vi "RT Loop - Acquire camera_data.vi"(11 "Message Queue":refnum<queue>) -> (3 "Refnum out":T1(plugin-control))   [LabVIEW 2017]
uses:
  UI Error Handlers/support/Message Queue/Message Cluster.ctl
  <vilib>/userdefined/High Color/IMAQdx.ctl
  <vilib>/vision/Avi.llb/IMAQ AVI2 Codec Path.ctl
  <vilib>/vision/Avi.llb/IMAQ AVI2 Refnum.ctl
  Globals/Global - All RT Loop Stop.vi
  Globals/Global - Configuration Options.vi
  <vilib>/vision/driver/NI_Vision_Acquisition_Software.lvlib
  UI Error Handlers/support/Message Queue/Message Queue.lvlib
panel:
  out "Acceleration Log Folder":path=path "/home/lvuser/Log/logfiles_deploy"
  out "Codec Names":string[](array[string])
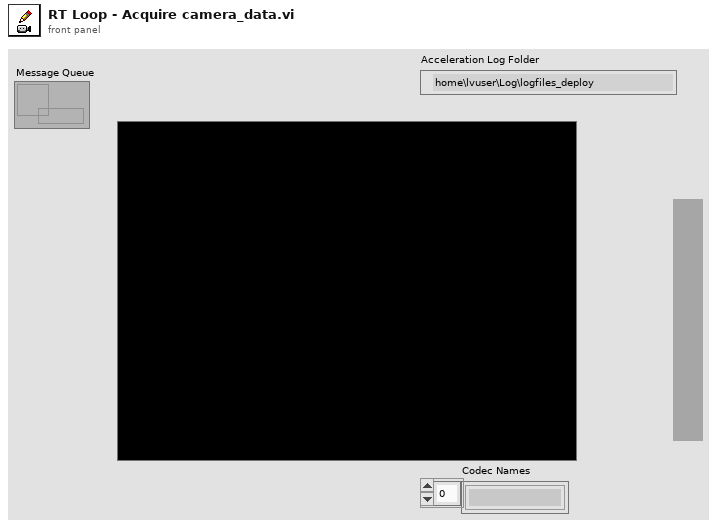
[diagram p1: front panel]
types:
  T1 = typedef "IMAQ Image.ctl" = refnum<image>
  T2 = typedef "IMAQdx.ctl" = refnum<k21>
  T3 = typedef "Image Type" = u32
  T4 = typedef "IMAQ AVI2 Refnum.ctl" = refnum<k20>
  T5 = typedef "IMAQ AVI2 Codec Path.ctl" = u32
  T6 = cluster{"Tool data":cluster{"Number of teeth":sgl}, "Cutting data":cluster{"rpm":sgl}, "Limits":cluster{"Magnitude threshold":sgl, "Tolerance":sgl}, "G1 status":cluster{"G1 trigger":bool}}
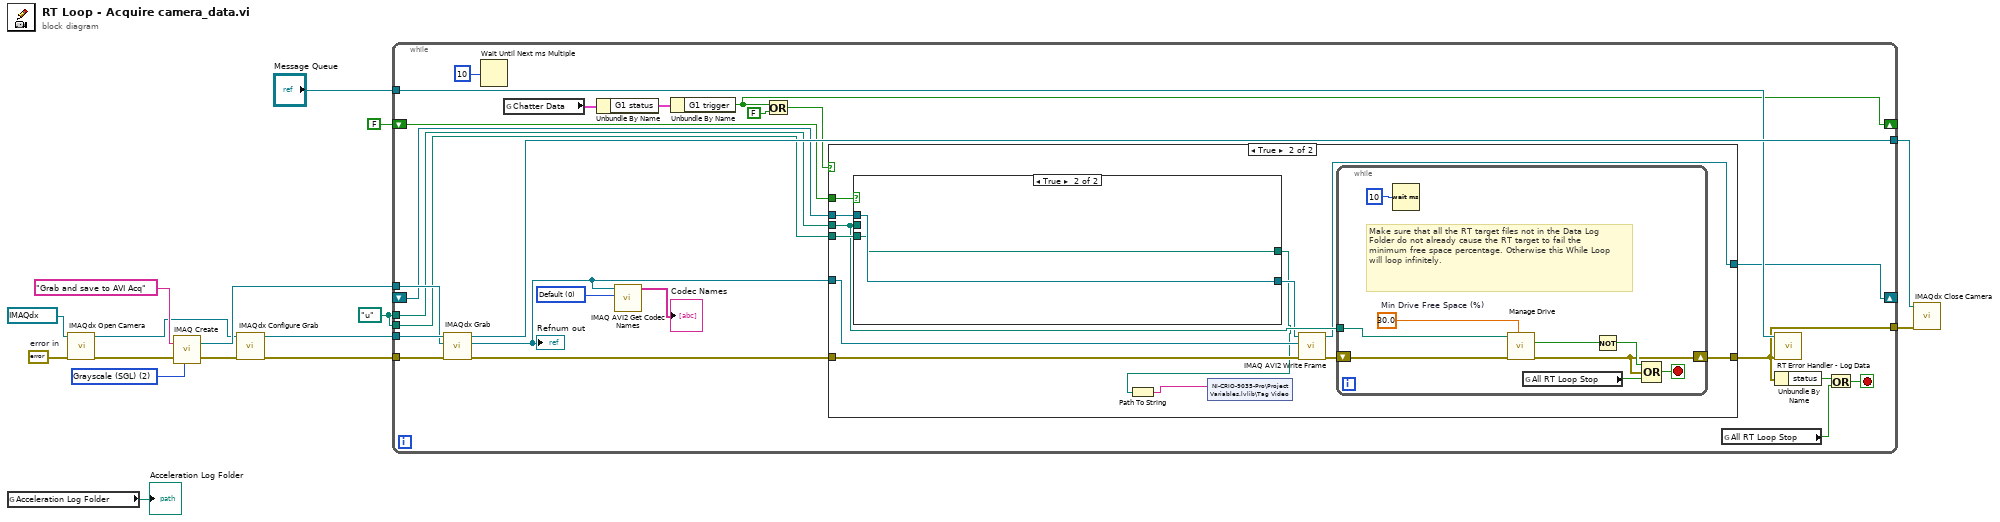
[diagram p0: block diagram]
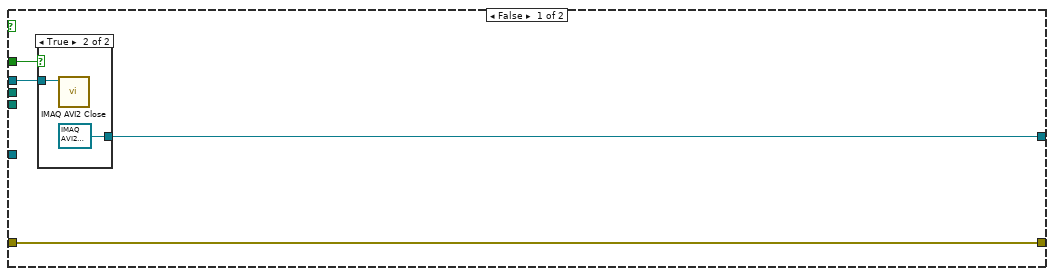
[diagram p2: hidden frame]
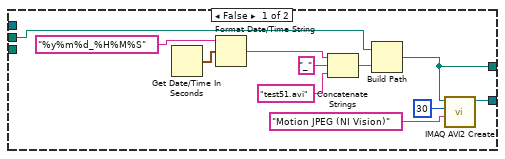
[diagram p4: hidden frame]
diagram:
  w2 = path "u:/" ("AVI Path")
  w12 = T3 2 items=["Grayscale (U8)", "Grayscale (I16)", "Grayscale (SGL)", "Complex (CSG)", "RGB (U32)", "HSL (U32)", "RGB (U64)", "Grayscale (U16)"] ("Image Type")
  w10 = errorcluster {"status"=FALSE, "code"=0, "source"=""}  # error in
  n1 = global read "Global - Configuration Options.vi" "Acceleration Log Folder"() -> (→"Acceleration Log Folder":path)
  n2 = call <vilib>:"IMAQdx Open Camera.vi"("error in"=w10, "Session In"=T2 "cam0") -> ("error out"=w13:errorcluster, "Session Out"=w8:T2)  [unwired: 8 in]
  n3 = call "IMAQ Create"("Image Name"="Grab and save to AVI Acq", "Image Type"=w12, "error in (no error)"=w13) -> ("New Image"=w16:T1, "error out"=w1:errorcluster)  [unwired: 2 in]
  n4 = call <vilib>:"IMAQdx Configure Grab.vi"("error in"=w1, "Session In"=w8) -> ("error out"=w15:errorcluster, "Session Out"=w14:T2)  [unwired: 8 in]
  n5 = while {
    tunnel: w15 -> [w40]
    tunnel: w14 -> [w39]
    tunnel: w16 -> [w38]
    tunnel: [w26] -> w6
    tunnel: [w37] -> w7
    tunnel: w2 -> [w29]
    tunnel: "Message Queue" -> [w27]
    tunnel: w2 -> [w21]
    shift-right: [w18] -> _
    shift-left: _ -> [w17]
    shift-right: [w20] -> _
    shift-left: FALSE ("G1 trigger") -> [w19]
    stop <- w34 stop-if-true
    w33 = T5 0 items=["Default", "System", "Built in Vision"] ("Codec Source")
    n6 = call <vilib>:"IMAQdx Grab.vi"("error in"=w40, "Image In"=w38, "Session In"=w39) -> ("error out"=w30:errorcluster, "Image Out"=w31:T1, "Session Out"=w37:T2)  [unwired: 5 in, 1 out]
    "Refnum out" <- w31
    n7 = Wait Until Next ms Multiple(millisecond multiple=u32 10 ("milliseconds to wait")) -> ()  [unwired: 1 out]
    n8 = global read "Global - Configuration Options.vi" "Chatter Data"() -> (w25:T6)
    n9 = Unbundle By Name(w25) -> ("G1 status"=w24:cluster{"G1 trigger":bool})
    n10 = call "IMAQ AVI2 Get Codec Names"("Codec Source"=w33, "Image"=w31) -> ("Codec Names"=→"Codec Names":string[])  [unwired: 8 in, 1 out]
    n11 = Unbundle By Name(w24) -> ("G1 trigger"=w20:bool)
    n12 = Or(x=w20, y=FALSE) -> (x .or. y?=w22:bool)
    n13 = case shown="True" w22 {
      tunnel: w31 -> [_ w54]
      tunnel: w30 -> [w44 w50]
      tunnel: [w44 w59] -> w26
      tunnel: w29 -> [_ w57]
      tunnel: w21 -> [_ w58]
      tunnel: w19 -> [w42 w56]
      tunnel: [w41 w52] -> w18
      tunnel: w17 -> [w43 w51]
      frame False {
        n14 = case shown="True" w42 {
          tunnel: w43 -> [w45 w47]
          tunnel: [w45 T4 refnum ("AVI Refnum (duplicate)")] -> w41
          frame False {
          }
          frame True {
            n15 = call "IMAQ AVI2 Close"("AVI Refnum"=w47) -> ()  [unwired: 10 in, 1 out]
          }
        }
      }
      frame True {
        n16 = case shown="True" w56 {
          tunnel: w58 -> [_ w71]
          tunnel: w57 -> [w64 _]
          tunnel: [w61 w72] -> w55
          tunnel: w51 -> [_ w72]
          tunnel: [w60 w71] -> w49
          frame False {
            n17 = Get Date/Time In Seconds() -> (seconds since 1Jan1904=w66:timestamp)
            n18 = Format Date/Time String(time format string (%c)="%y%m%d_%H%M%S", seconds (now)=w66) -> (date/time string=w67:string)  [unwired: 1 out]
            n19 = Concatenate Strings(w67, "_" ("string"), "test51.avi" ("name or relative path")) -> (w70:string)
            n20 = Build Path(base path=w64, name or relative path=w70) -> (appended path=w60:path)
            n21 = call "IMAQ AVI2 Create"("Codec"="Motion JPEG (NI Vision)", "Frames Per Second"=u32 30, "AVI Path"=w60) -> ("AVI Refnum"=w61:T4)  [unwired: 7 in, 1 out]
          }
          frame True {
          }
        }
        n22 = Path To String(path=w49) -> (string=w48:string)
        n23 = shared-variable "NI-CRIO-9035-Pro\\Project Variables.lvlib\\Tag Video"(w48) -> ()  [unwired: 1 in, 1 out]
        n24 = call "IMAQ AVI2 Write Frame"("error in (no error)"=w50, "Image"=w54, "AVI Refnum"=w55) -> ("error out"=w53:errorcluster, "AVI Refnum (duplicate)"=w52:T4)  [unwired: 6 in, 1 out]
        n25 = while {
          shift-right: [w76] -> w59
          shift-left: w53 -> [w77]
          tunnel: w57 -> [w74]
          stop <- w81 stop-if-true
          w75 = 30.0  # Min Drive Free Space (%)
          # "Make sure that all the RT target files not in the Data Log Folder do not already cause the RT target to fail the minimum free space percentage. Otherwise this While Loop will loop infinitely."
          n26 = Wait (ms)(milliseconds to wait=u32 10) -> ()  [unwired: 1 out]
          n27 = call "Manage Drive.vi"("Min Drive Free Space (%)"=w75, "error in"=w77, "Data Folder"=w74) -> ("error out"=w76:errorcluster, "Drive Space Below Limit"=w73:bool)  [unwired: 7 in]
          n28 = global read "Global - All RT Loop Stop.vi" "All RT Loop Stop"() -> (w78:bool)
          n29 = Not(x=w73) -> (.not. x?=w80:bool)
          n30 = Compound Arithmetic op=OR(w80, w76, w78) -> (w81:bool)
        }
      }
    }
    n31 = global read "Global - All RT Loop Stop.vi" "All RT Loop Stop"() -> (w28:bool)
    n32 = call "RT Error Handler - Log Data.vi"("error in (no error)"=w26, "Message Queue"=w27) -> ()  [unwired: 9 in, 1 out]
    n33 = Unbundle By Name(w26) -> ("status"=w35:bool)
    n34 = Or(x=w35, y=w28) -> (x .or. y?=w34:bool)
  }
  n35 = call <vilib>:"IMAQdx Close Camera.vi"("error in"=w6, "Session In"=w7) -> ()  [unwired: 9 in, 1 out]
